vi "Sequence.CreateWhileLoop.vi"(8 "error in (no error)":errorcluster, 10 "Expression":string, 11 "Task Ref":refnum<k24>) -> (0 "error out":errorcluster, 3 "Task Ref out":refnum<k24>)   [LabVIEW 2015, in "Single Station Execution.lvlib"]
uses:
  Single Station Execution.lvlib
  NationalInstruments.VeriStand.RealTimeSequenceDefinitionApi
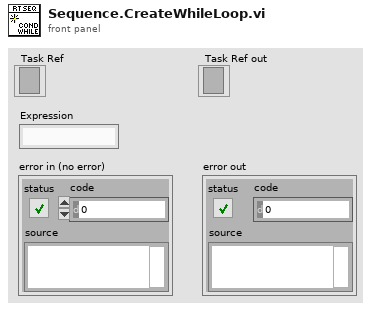
[diagram p1: front panel]
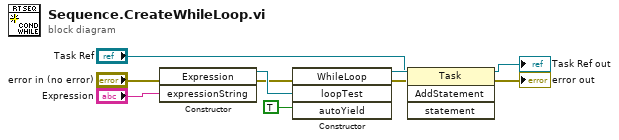
[diagram p0: block diagram]
diagram:
  n1 = constructor class="Expression"(error in="error in (no error)", "expressionString"="Expression") -> (reference out=w2:refnum<k24>, error out=w1:errorcluster)  [unwired: 2 in, 2 out]
  n2 = constructor class="WhileLoop"(error in=w1, "loopTest"=w2, "autoYield"=TRUE) -> (reference out=w8:refnum<k24>, error out=w7:errorcluster)  [unwired: 2 in, 3 out]
  n3 = invoke class="Task" method="AddStatement"(reference="Task Ref", error in=w7, "statement"=w8) -> (reference out=→"Task Ref out":refnum<k24>, error out=→"error out":errorcluster)  [unwired: 1 in, 2 out]
